vi "Set Counter.vi"(8 "error in (no error)":errorcluster, 10 "Input":dbl, 11 "Feeder Actor.lvlib:Counter.lvclass":refnum<class "Counter.lvclass">) -> (0 "error out":errorcluster, 3 "Feeder Actor.lvlib:Counter.lvclass":refnum<class "Counter.lvclass">)   [LabVIEW 2018, in "Feeder Actor.lvlib" / "Counter.lvclass"]
uses:
  Counter.lvclass
  Counter.lvclass/Counter.ctl
  <resource>/objmgr/daqmx.rc
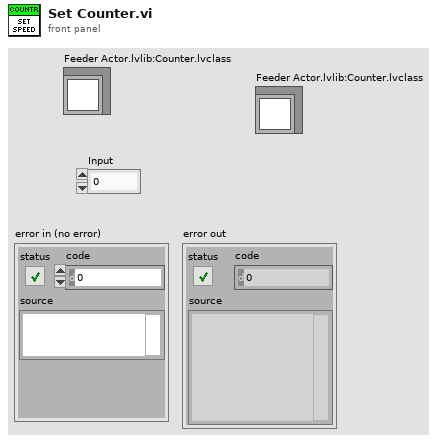
[diagram p1: front panel]
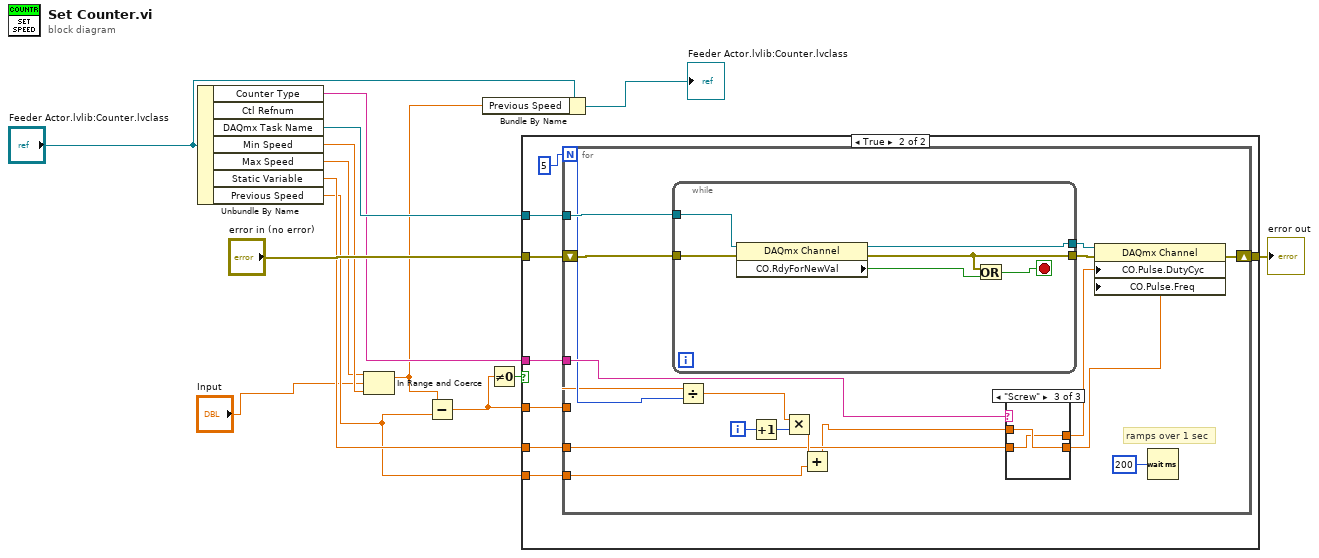
[diagram p0: block diagram]
diagram:
  n1 = Unbundle By Name("Feeder Actor.lvlib:Counter.lvclass") -> ("Counter Type"=w10:string, "DAQmx Task Name"=w12:refnum<k21>, "Min Speed"=w9:dbl, "Max Speed"=w8:dbl, "Static Variable"=w7:dbl, "Previous Speed"=w3:dbl)  [unwired: 1 out]
  n2 = In Range and Coerce(upper limit=w8, x="Input", lower limit=w9) -> (coerced(x)=w6:dbl)  [unwired: 1 out]
  n3 = Subtract(x=w6, y=w3) -> (x-y=w4:dbl)
  n4 = Bundle By Name(cluster="Feeder Actor.lvlib:Counter.lvclass", "Previous Speed"=w6) -> (→"Feeder Actor.lvlib:Counter.lvclass":refnum<class "Counter.lvclass">)
  n5 = Not Equal To 0?(x=w4) -> (x != 0?=w5:bool)
  n6 = case shown="True" w5 {
    tunnel: [w15 w23] -> w14
    tunnel: "error in (no error)" -> [w15 w22]
    tunnel: w12 -> [_ w21]
    tunnel: w10 -> [_ w20]
    tunnel: w7 -> [_ w19]
    tunnel: w4 -> [_ w18]
    tunnel: w3 -> [_ w16]
    frame False {
    }
    frame True {
      n7 = for {
        N: 5 -> [w32]
        tunnel: w21 -> [w39]
        tunnel: w20 -> [w36]
        tunnel: w19 -> [w26]
        shift-right: [w41] -> w23
        shift-left: w22 -> [w40]
        tunnel: w18 -> [w27]
        tunnel: w16 -> [w24]
        i -> [w30]
        # "ramps over 1 sec"
        n8 = while {
          tunnel: w40 -> [w53]
          tunnel: w39 -> [w52]
          tunnel: [w51] -> w38
          tunnel: [w49] -> w37
          stop <- w48 stop-if-true
          n9 = property class="DAQmx Channel"(reference=w52, error in=w53) -> (reference out=w51:refnum<k21>, error out=w49:errorcluster, "CO.RdyForNewVal"=w50:bool)
          n10 = Or(x=w49, y=w50) -> (x .or. y?=w48:bool)
        }
        n11 = Divide(x=w27, y=w32) -> (x/y=w31:dbl)
        n12 = Increment(x=w30) -> (x+1=w29:i32)
        n13 = Multiply(x=w31, y=w29) -> (x*y=w28:dbl)
        n14 = Add(x=w28, y=w24) -> (x+y=w25:dbl)
        n15 = case shown="\"Screw\"" w36 {
          tunnel: w25 -> [w43 w45 w47]
          tunnel: [w42 w44 w47] -> w35
          tunnel: [w43 w45 w46] -> w34
          tunnel: w26 -> [w42 w44 w46]
          frame "False", Default {
          }
          frame "Mixer" {
          }
          frame "Screw" {
          }
        }
        n16 = property class="DAQmx Channel"(reference=w38, error in=w37, "CO.Pulse.DutyCyc"=w34, "CO.Pulse.Freq"=w35) -> (error out=w41:errorcluster)  [unwired: 1 out]
        n17 = Wait (ms)(milliseconds to wait=u32 200) -> ()  [unwired: 1 out]
      }
    }
  }
  "error out" <- w14
